vi "调用宏命令.vi"(8 "error in (no error)":errorcluster caption="错误输入（无错误）", 11 "控制盒（宏命令） 输入":refnum<class "控制盒（宏命令）.lvclass"> caption="DNL_LabVIEW Object in") -> (0 "error out":errorcluster caption="错误输出", 3 "控制盒（宏命令） 输出":refnum<class "控制盒（宏命令）.lvclass"> caption="DNL_LabVIEW Object out")   [LabVIEW 2011, in "控制盒（宏命令）.lvclass"]
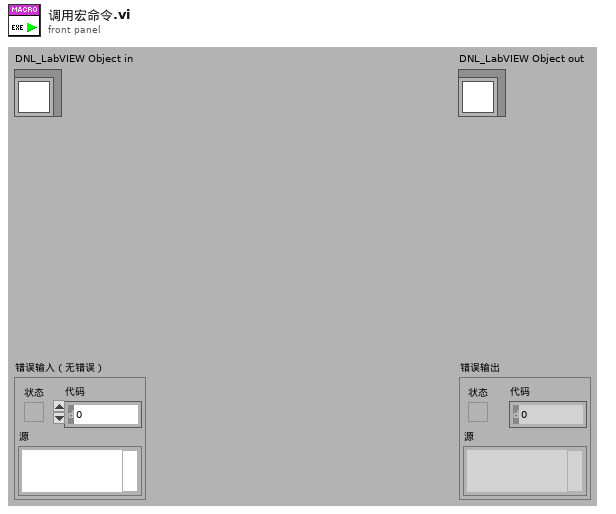
[diagram p1: front panel]
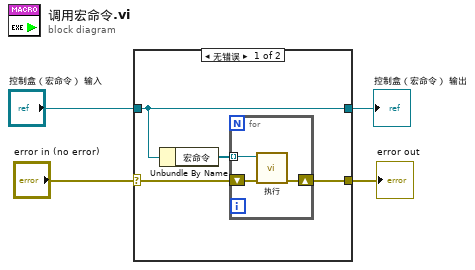
[diagram p0: block diagram]
diagram:
  n1 = case shown="无错误" "error in (no error)" {
    selector: "error in (no error)" -> [w6 w13]
    tunnel: [w5 w13] -> w3
    tunnel: [w8 w12] -> w1
    tunnel: "控制盒（宏命令） 输入" -> [w8 w12]
    frame No Error {
      n2 = Unbundle By Name(w8) -> ("宏命令"=w7:refnum<class "命令类.lvclass">[])
      n3 = for {
        tunnel: w7 -> [w11] mode=indexing
        shift-right: [w9] -> w5
        shift-left: w6 -> [w10]
        n4 = call-dynamic "执行.vi"("error in (no error)"=w10, "命令类 输入"=w11) -> ("error out"=w9:errorcluster)  [unwired: 8 in, 1 out]
      }
    }
    frame Error {
    }
  }
  "error out" <- w3
  "控制盒（宏命令） 输出" <- w1
